vi "append filename.vi"(10 "string":string=" - running averages", 11 "path":path) -> (3 "path 2":path)   [LabVIEW 2018]
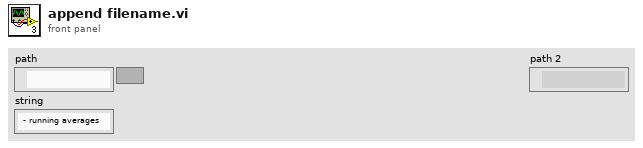
[diagram p1: front panel]
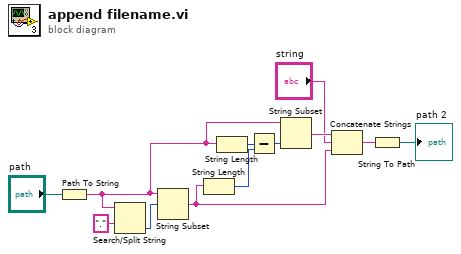
[diagram p0: block diagram]
diagram:
  n1 = Path To String(path="path") -> (string=w1:string)
  n2 = Search/Split String(string=w1, search string/char (-)=".") -> (offset of match=w4:i32)  [unwired: 1 in, 2 out]
  n3 = String Subset(string=w1, offset (0)=w4) -> (substring=w3:string)  [unwired: 1 in]
  n4 = String Length(string=w3) -> (length=w2:i32)
  n5 = String Length(string=w1) -> (length=w9:i32)
  n6 = Subtract(x=w9, y=w2) -> (x-y=w10:i32)
  n7 = String Subset(string=w1, length (rest)=w10) -> (substring=w12:string)  [unwired: 1 in]
  n8 = Concatenate Strings(w12, "string", w3) -> (w11:string)
  n9 = String To Path(string=w11) -> (path=→"path 2":path)
